vi "cluster exercise.vi"() -> ()   [LabVIEW 2016]
panel:
  out "String":string
  in  "stop":bool
  out "Output Cluster":T1
  in  "Input Cluster":T1
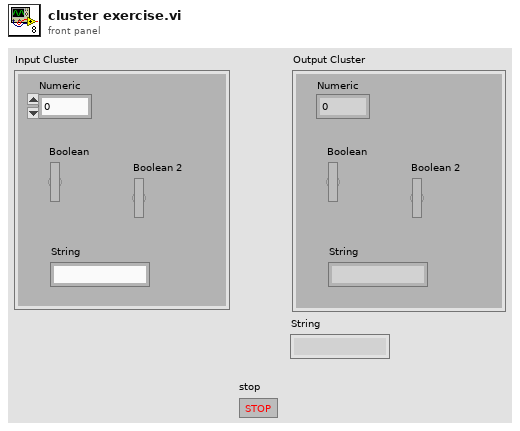
[diagram p1: front panel]
types:
  T1 = cluster{"Numeric":dbl, "Boolean":bool, "Boolean 2":bool, "String":string}
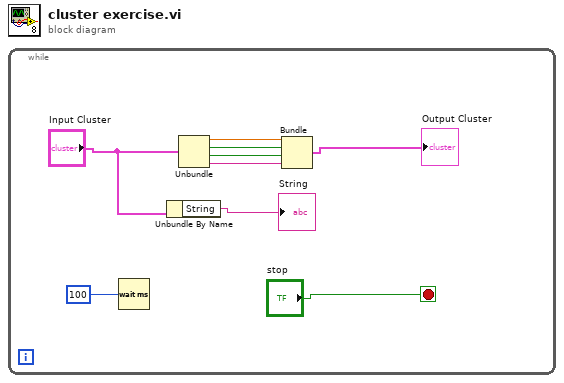
[diagram p0: block diagram]
diagram:
  n1 = while {
    stop <- "stop" stop-if-true
    n2 = Wait (ms)(milliseconds to wait=u32 100 ("millisecond timer value")) -> ()  [unwired: 1 out]
    n3 = Unbundle By Name("Input Cluster") -> ("String"=→"String":string)
    n4 = Unbundle "Unbundle"("Input Cluster") -> ("Numeric"=w8:dbl, "Boolean"=w7:bool, "Boolean 2"=w6:bool, "String"=w5:string)
    n5 = Bundle "Bundle"("Numeric"=w8, "Boolean"=w7, "Boolean 2"=w6, "String"=w5) -> (→"Output Cluster":T1)  [unwired: 1 in]
  }
